vi "PDLM_GetLHVersion.vi"(8 "error in (no error)":errorcluster, 11 "USBIdx":i32) -> (0 "error out":errorcluster, 2 "Version":string, 3 "return type":i32)   [LabVIEW 2019]
uses:
  <userlib>/TaikoLaser/PDLM_DllPath_global.vi
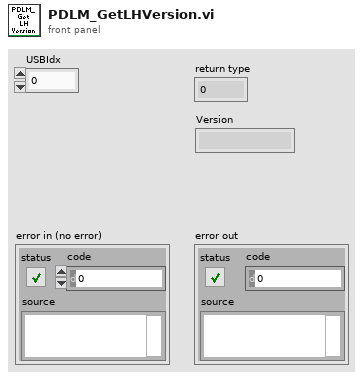
[diagram p1: front panel]
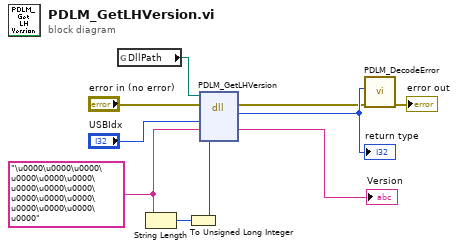
[diagram p0: block diagram]
diagram:
  w3 = "\u0000\u0000\u0000\u0000\u0000\u0000\u0000\u0000\u0000\u0000\u0000\u0000\u0000\u0000\u0000\u0000" ("Version")
  n1 = global read "PDLM_DllPath_global.vi" "DllPath"() -> (w6:path)
  n2 = String Length(string=w3) -> (length=w4:i32)
  n3 = To Unsigned Long Integer(number=w4) -> (unsigned 32bit integer=w2:u32)
  n4 = dll-call lib="M:/_dev/progs/LabVIEW/_lib/PQ/Taiko/pdlm_lib.dll" fn="PDLM_GetLHVersion"(path in=w6, error in="error in (no error)", "USBIdx"="USBIdx", "Version"=w3, "BuffLen"=w2) -> (error out=w8:errorcluster, "return type"=w9:i32, "Version"=→"Version":string)  [unwired: 3 in, 1 out]
  "return type" <- w9
  n5 = call <userlib>:"PDLM_DecodeError.vi"("error in (no error)"=w8, "code"=w9) -> ("error out"=→"error out":errorcluster)  [unwired: 7 in, 2 out]
